vi "Main.vi"() -> ()   [LabVIEW 2019, in "Money.lvlib"]
doc: "This template is based off of the Queued Message Handler design pattern and the Queued Message Handler project template that ships with LabVIEW.\n\nThe main difference is that the queue is private to this module and communication between modules is performed via Broadcast and Request events.\n\nRequest events are wrapped in public API methods and are handled in the Event Handling Loop (EHL) of this VI. Any module can register for Broadcast events sent by this module. The EHL generates messages based on user interface actions.\n\nThe Message Handling Loop (MHL) processes messages generated by the EHL, or by other messages. The messages are string values, so new messages can be added easily to the Message Cases case structure in the MHL. Each message cluster can also provide an optional value for Message Data, which is a variant that can be converted to whatever message-specific data is required.\n_____\nBased on Delacor QMH Project Template 4.2.1.64."
uses:
  Money.lvlib
  <vilib>/Delacor/Delacor QMH/Libraries/Module Admin_class/Delacor_lib_QMH_Module Admin.lvclass
  Module Data--cluster.ctl
  <vilib>/Delacor/Delacor QMH/Libraries/Message Queue_class/Delacor_lib_QMH_Message Queue.lvclass/Delacor_lib_QMH_Message Queue.ctl
  Stop Argument--cluster.ctl
  <vilib>/Delacor/Delacor QMH/Libraries/Module Admin_class/Delacor_lib_QMH_Module Admin.lvclass/Delacor_lib_QMH_Module Admin.ctl
  Add to Balance Argument--cluster.ctl
  Add to Balance (Reply Payload)--cluster.ctl
  Refund Money Argument--cluster.ctl
  Check Funds Argument--cluster.ctl
  Check Funds (Reply Payload)--cluster.ctl
  Reduce Funds Argument--cluster.ctl
  Reduce Funds (Reply Payload)--cluster.ctl
  <vilib>/Utility/miscctls.llb/LVPointTypeDef.ctl
  <vilib>/Delacor/Delacor QMH/Libraries/Message Queue_class/Delacor_lib_QMH_Enqueue Message (Single).vi
  <vilib>/Delacor/Delacor QMH/Libraries/Module Admin_class/Delacor_lib_QMH_Get External Launch.vi
  <vilib>/Utility/error.llb/Error Cluster From Error Code.vi
  <vilib>/ErrorRing/Error Ring.xnode
  <vilib>/Delacor/Delacor QMH/Libraries/Message Queue_class/Delacor_lib_QMH_Message Queue.lvclass
panel:
  in  "Subpanel Ref":refnum<vi>
  in  "Money":T1
  in  "Simulate MHL Error":bool
  in  "Simulate EHL Error":bool
  out "error out":errorcluster
  in  "Module Admin":refnum<class "Delacor_lib_QMH_Module Admin.lvclass">
  out "Status":string
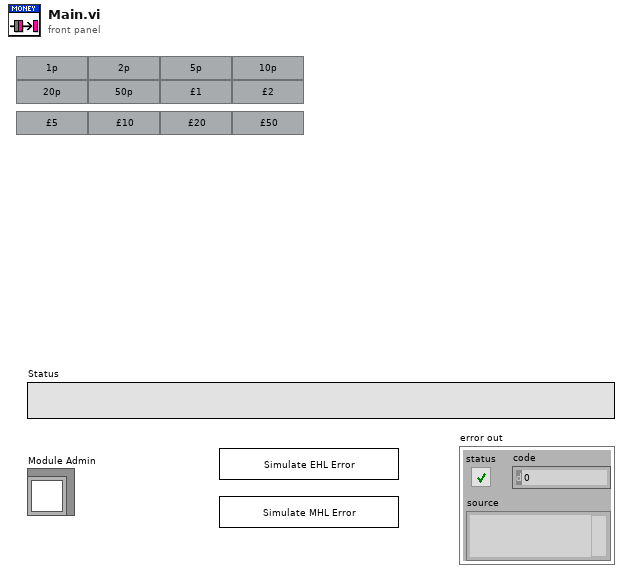
[diagram p1: front panel]
types:
  T1 = cluster{"1":bool, "2":bool, "5":bool, "10":bool, "20":bool, "50":bool, "100":bool, "200":bool, "500":bool, "1000":bool, "2000":bool, "5000":bool}
  T2 = typedef "Money.lvlib/Request Events--cluster.ctl" = cluster{"Stop Module":refnum<user-event>, "Show Panel":refnum<user-event>, "Hide Panel":refnum<user-event>, "Get Module Execution Status":refnum<user-event>, "Show Diagram":refnum<user-event>, "Refund Money":refnum<user-event>, "Check Funds":refnum<user-event>, "Reduce Funds":refnum<user-event>, "Add to Balance":refnum<user-event>}
  T3 = typedef "Money.lvlib/Module Data--cluster.ctl" = cluster{"Status":string, "Balance (pence)":u32}
  T4 = enum32{"invalid lock state", "Not Locked", "Locked (No Password)", "Password-protected"}
  T5 = typedef "Money.lvlib/Stop Argument--cluster.ctl" = cluster{"Origin":string, "Exit via Stop Module Req?":bool, "Wait for Module to stop?":bool}
  T6 = typedef "Money.lvlib/Add to Balance Argument--cluster.ctl" = cluster{"Balance to add":u32, "Wait Notifier":refnum<notifier>, "wait for reply":bool}
  T7 = typedef "Money.lvlib/Refund Money Argument--cluster.ctl" = cluster{"Boolean":bool}
  T8 = typedef "Money.lvlib/Check Funds Argument--cluster.ctl" = cluster{"Minimum Amount":u32, "Wait Notifier":refnum<notifier>, "wait for reply":bool}
  T9 = typedef "Money.lvlib/Reduce Funds Argument--cluster.ctl" = cluster{"Reduce Funds":i32, "Wait Notifier":refnum<notifier>, "wait for reply":bool}
  T10 = typedef "LVPointTypeDef.ctl" = cluster{"Horizontal":i16, "Vertical":i16}
  T11 = typedef "Money.lvlib/Check Funds (Reply Payload)--cluster.ctl" = cluster{"Sufficient Funds":bool, "Check Funds_error":errorcluster, "Balance":u32}
  T12 = typedef "Money.lvlib/Reduce Funds (Reply Payload)--cluster.ctl" = cluster{"Remaining Balance":u32, "Reduce Funds_error":errorcluster, "Sucessful":bool}
  T13 = typedef "Money.lvlib/Add to Balance (Reply Payload)--cluster.ctl" = cluster{"Add to Balance_error":errorcluster, "New Balance":u32}
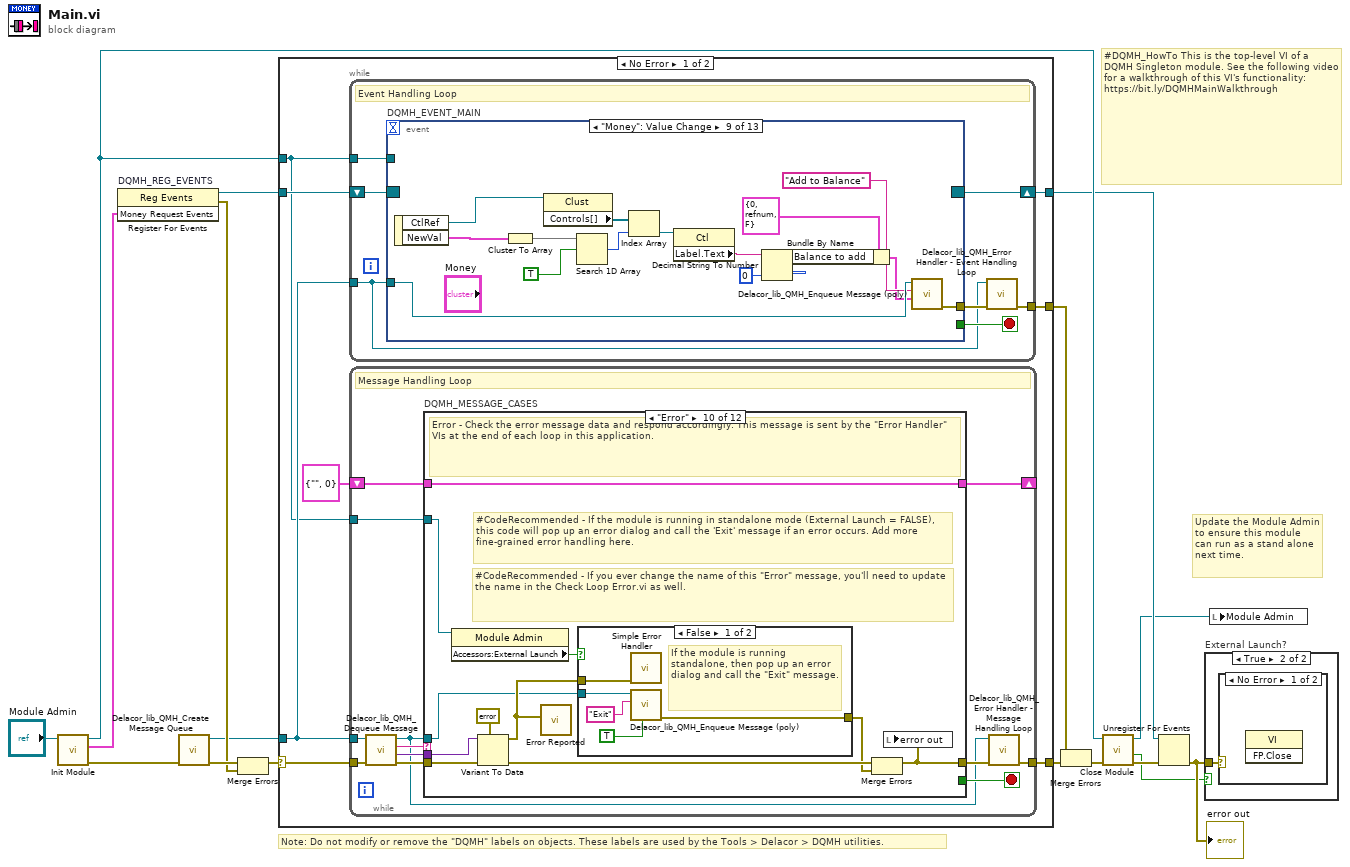
[diagram p0: block diagram]
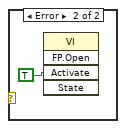
[diagram p3: hidden frame]
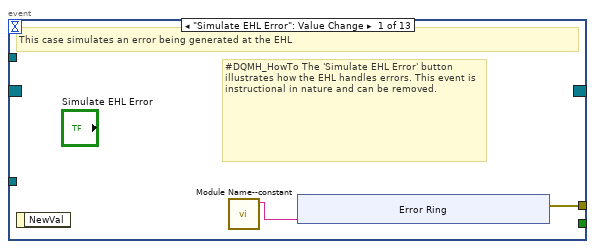
[diagram p4: hidden frame]
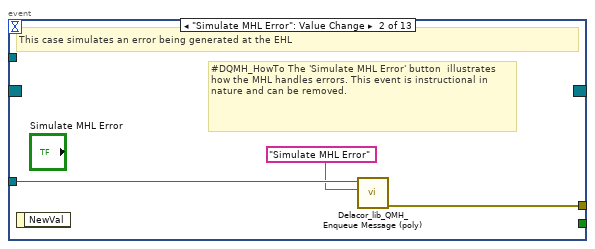
[diagram p5: hidden frame]
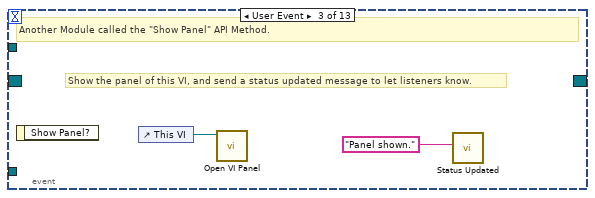
[diagram p6: hidden frame]
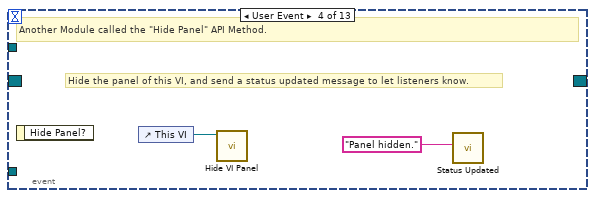
[diagram p7: hidden frame]
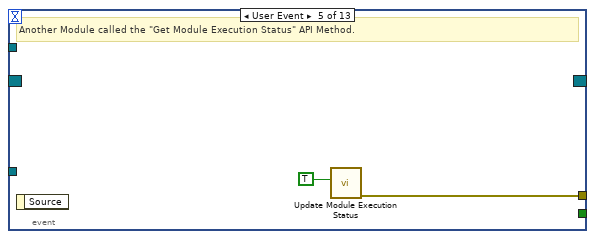
[diagram p8: hidden frame]
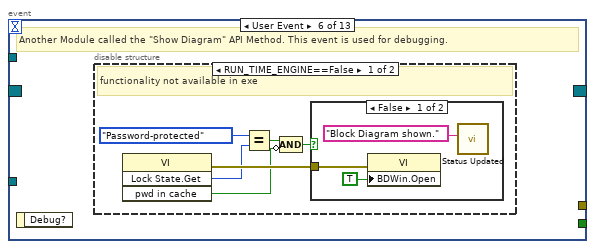
[diagram p9: hidden frame]
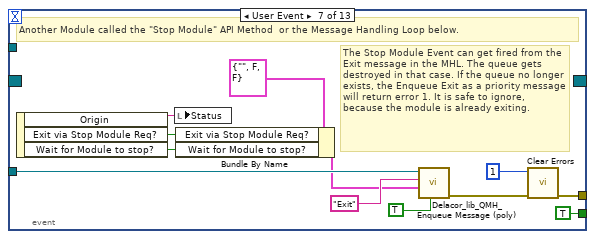
[diagram p12: hidden frame]
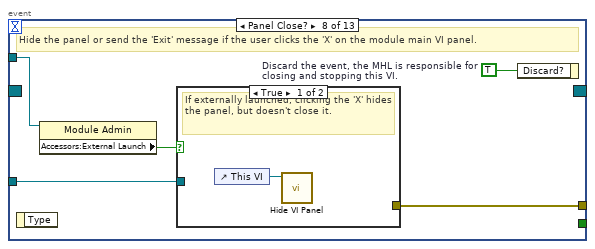
[diagram p13: hidden frame]
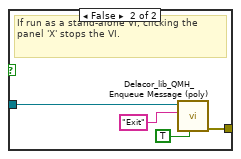
[diagram p14: hidden frame]
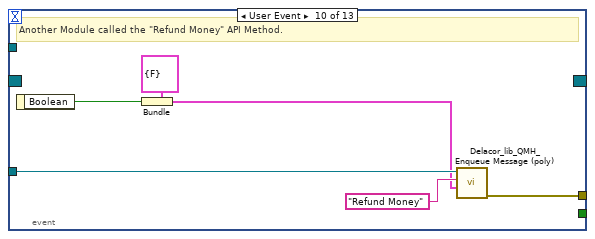
[diagram p15: hidden frame]
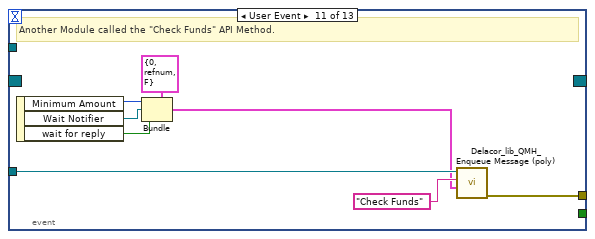
[diagram p16: hidden frame]
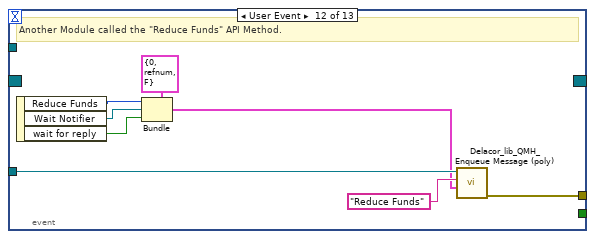
[diagram p17: hidden frame]
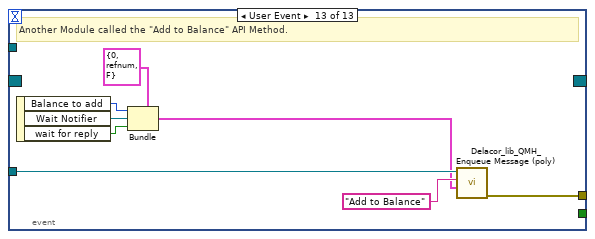
[diagram p18: hidden frame]
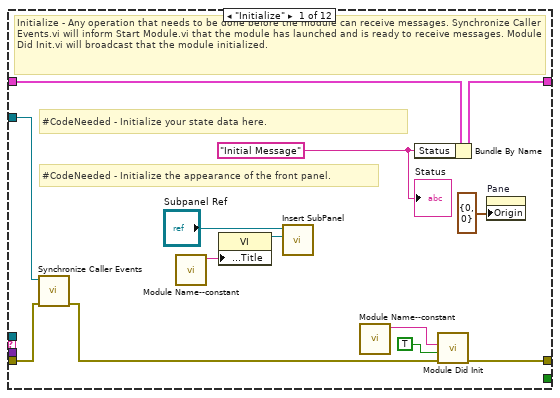
[diagram p19: hidden frame]
diagram:
  # "#DQMH_HowTo This is the top-level VI of a DQMH Singleton module. See the following video for a walkthrough of this VI's functionality: https://bit.ly/DQMHMainWalkthrough"
  # "Note: Do not modify or remove the \"DQMH\" labels on objects. These labels are used by the Tools > Delacor > DQMH utilities."
  # "Update the Module Admin to ensure this module can run as a stand alone next time."
  n1 = call "Init Module.vi"("Singleton Module Admin in"="Module Admin") -> ("error out"=w16:errorcluster, "Money Request Events"=w5:T2, "Singleton Module Admin out"=w8:refnum<class "Delacor_lib_QMH_Module Admin.lvclass">)  [unwired: 8 in]
  n2 = register-events "DQMH_REG_EVENTS"(w5) -> (reference out=w6:refnum<event-registration>, error out=w9:errorcluster)  [unwired: 2 in]
  n3 = call <vilib>:"Delacor_lib_QMH_Create Message Queue.vi"("error in (no error)"=w16) -> ("error out"=w11:errorcluster, "Message Queue"=w4:refnum<class "Delacor_lib_QMH_Message Queue.lvclass">)  [unwired: 9 in]
  n4 = Merge Errors(w11, w9) -> (w10:errorcluster)
  n5 = case shown="No Error" w10 {
    selector: w10 -> [w23 w292]
    tunnel: [w25 w292] -> w17
    tunnel: [w22 w289] -> w7
    tunnel: w6 -> [w20 w289]
    tunnel: w4 -> [w19 _]
    tunnel: [w24 _] -> w14
    tunnel: w8 -> [w18 w285]
    frame No Error {
      n6 = while {
        tunnel: w19 -> [w26]
        shift-right: [w29] -> w22
        shift-left: w20 -> [w30]
        tunnel: [w31] -> w24
        tunnel: w18 -> [w27]
        stop <- w28 stop-if-true
        # "Event Handling Loop"
        n7 = event "DQMH_EVENT_MAIN" shown="[8] \"Money\": Value Change" {
          selector: w30 -> [_ _ _ _ _ _ _ _ _ _ _ _ _]
          dyn-events: [_ _ _ _ _ _ _ _ _ _ _ _ _] -> w29
          timeout: _ -> [_ _ _ _ _ _ _ _ _ _ _ _ _]
          tunnel: [_ _ _ _ _ _ TRUE ("Discard?") _ _ _ _ _ _] -> w28
          tunnel: w26 -> [_ w43 _ _ _ _ w67 w74 w86 w102 w110 w118 w126]
          tunnel: [w34 w44 _ _ w50 _ w70 w76 w87 w97 w103 w111 w124] -> w32
          tunnel: w27 -> [_ _ _ _ _ _ _ w73 _ _ _ _ _]
          event "Simulate EHL Error": Value Change {
            # "#DQMH_HowTo The 'Simulate EHL Error' button  illustrates how the EHL handles errors. This event is instructional in nature and can be removed."
            # "This case simulates an error being generated at the EHL"
            n8 = event-data() -> ()  [unwired: 1 in, 1 out]
            n9 = call "Module Name--constant.vi"() -> ("Module Name"=w33:string)  [unwired: 11 in]
            n10 = xnode "Error Ring"("parameter 0"=w33) -> ("error out"=w34:errorcluster)
          }
          event "Simulate MHL Error": Value Change {
            # "#DQMH_HowTo The 'Simulate MHL Error' button  illustrates how the MHL handles errors. This event is instructional in nature and can be removed."
            # "This case simulates an error being generated at the EHL"
            n11 = event-data() -> ()  [unwired: 1 in, 1 out]
            n12 = call-poly <vilib>:"Delacor_lib_QMH_Enqueue Message (poly).vi"("Message"="Simulate MHL Error", "Message Queue in"=w43) -> ("error out"=w44:errorcluster)  [unwired: 8 in, 1 out]
          }
          event User Event {
            # "Show the panel of this VI, and send a status updated message to let listeners know."
            # "Another Module called the \"Show Panel\" API Method."
            n13 = event-data() -> ()  [unwired: 1 in, 1 out]
            n14 = control-ref of="This VI"() -> (w46:refnum<vi>)
            n15 = call "Open VI Panel.vi"("VI"=w46) -> ()  [unwired: 10 in, 1 out]
            n16 = call "Status Updated.vi"("Status"="Panel shown." ("format string")) -> ()  [unwired: 10 in, 1 out]
          }
          event User Event {
            # "Hide the panel of this VI, and send a status updated message to let listeners know."
            # "Another Module called the \"Hide Panel\" API Method."
            n17 = event-data() -> ()  [unwired: 1 in, 1 out]
            n18 = control-ref of="This VI"() -> (w48:refnum<vi>)
            n19 = call "Hide VI Panel.vi"("VI"=w48) -> ()  [unwired: 10 in, 1 out]
            n20 = call "Status Updated.vi"("Status"="Panel hidden." ("format string")) -> ()  [unwired: 10 in, 1 out]
          }
          event User Event {
            # "Another Module called the \"Get Module Execution Status\" API Method."
            n21 = event-data() -> ()  [unwired: 1 in, 1 out]
            n22 = call "Update Module Execution Status.vi"("Running?"=TRUE) -> ("error out"=w50:errorcluster)  [unwired: 10 in]
          }
          event User Event {
            # "Another Module called the \"Show Diagram\" API Method. This event is used for debugging."
            n23 = event-data() -> ()  [unwired: 1 in, 1 out]
            n24 = disable-structure shown="RUN_TIME_ENGINE==False" {
              frame condition #0 (active) {
                # "functionality not available in exe"
                n25 = invoke class="VI" method="Lock State.Get"() -> (error out=w56:errorcluster, "Get Lock State"=w55:T4, "pwd in cache"=w52:bool)  [unwired: 4 in, 1 out]
                n26 = Equal?(x=T4."Password-protected", y=w55) -> (x = y?=w53:bool)
                n27 = Compound Arithmetic op=AND(w53, invert w52) -> (w51:bool)
                n28 = case shown="False" w51 {
                  tunnel: w56 -> [w59 _]
                  frame False {
                    n29 = property class="VI"(error in=w59, "BDWin.Open"=TRUE ("Block Diagram Window:Open")) -> ()  [unwired: 1 in, 2 out]
                    n30 = call "Status Updated.vi"("Status"="Block Diagram shown." ("format string")) -> ()  [unwired: 10 in, 1 out]
                  }
                  frame True {
                    # "Password-protected VI, and the password is not in the cache. Do not show the diagram."
                  }
                }
              }
              frame condition #1 {
              }
            }
          }
          event User Event {
            # "The Stop Module Event can get fired from the Exit message in the MHL. The queue gets destroyed in that case. If the queue no longer exists, the Enqueue Exit as a priority message will return error 1. It is safe to ignore, because the module is already exiting."
            # "Another Module called the \"Stop Module\" API Method  or the Message Handling Loop below."
            n31 = event-data() -> ("Origin"=w66:string, "Exit via Stop Module Req?"=w62:bool, "Wait for Module to stop?"=w61:bool)  [unwired: 1 in]
            n32 = local write "Status"(w66) -> ()
            n33 = Bundle By Name(cluster=T5 {"Origin"="", "Exit via Stop Module Req?"=FALSE, "Wait for Module to stop?"=FALSE} ("Stop Argument"), "Exit via Stop Module Req?"=w62, "Wait for Module to stop?"=w61) -> (w60:T5)
            n34 = call-poly <vilib>:"Delacor_lib_QMH_Enqueue Message (poly).vi"("Priority Message? (F)"=TRUE, "Message Data"=w60, "Message"="Exit", "Message Queue in"=w67) -> ("error out"=w71:errorcluster)  [unwired: 6 in, 1 out]
            n35 = call <vilib>:"Clear Errors.vi"("error in (no error)"=w71, "specific error code to clear (0: all)"=1) -> ("error out"=w70:errorcluster)  [unwired: 4 in, 1 out]
          }
          event Panel Close? {
            w75 = TRUE  # Discard the event, the MHL is responsible for closing and stopping this VI.
            # "Hide the panel or send the 'Exit' message if the user clicks the 'X' on the module main VI panel."
            n36 = event-data() -> ()  [unwired: 1 in, 1 out]
            n37 = property class="Module Admin"(reference=w73) -> ("Accessors:External Launch"=w72:bool)  [unwired: 1 in, 2 out]
            n38 = case shown="True" w72 {
              tunnel: w74 -> [_ w80]
              tunnel: [_ w81] -> w76
              frame True {
                # "If externally launched, clicking the 'X' hides the panel, but doesn't close it."
                n39 = control-ref of="This VI"() -> (w77:refnum<vi>)
                n40 = call "Hide VI Panel.vi"("VI"=w77) -> ()  [unwired: 10 in, 1 out]
              }
              frame False {
                # "If run as a stand-alone VI, clicking the panel 'X' stops the VI."
                n41 = call-poly <vilib>:"Delacor_lib_QMH_Enqueue Message (poly).vi"("Priority Message? (F)"=TRUE, "Message"="Exit", "Message Queue in"=w80) -> ("error out"=w81:errorcluster)  [unwired: 7 in, 1 out]
              }
            }
            n42 = event-data("Discard?"=w75) -> ()  [unwired: 1 in, 1 out]
          }
          event "Money": Value Change {
            n43 = event-data() -> ("CtlRef"=w96:refnum<vi>, "NewVal"=w95:T1)  [unwired: 1 in]
            n44 = Cluster To Array(cluster=w95) -> (array=w94:bool[])
            n45 = property class="Clust"(reference=w96) -> ("Controls[]"=w88:refnum<vi>[])  [unwired: 1 in, 2 out]
            n46 = Search 1D Array(1D array=w94, element=TRUE) -> (index of element=w92:i32)  [unwired: 1 in]
            n47 = Index Array(array=w88, index=w92) -> (element=w91:refnum<vi>)
            n48 = property class="Ctl"(reference=w91) -> ("Label.Text"=w90:string)  [unwired: 1 in, 2 out]
            n49 = Decimal String To Number(string=w90, default (0L)=u32 0 ("default (0 I32)")) -> (number=w83:u32)  [unwired: 1 in, 1 out]
            n50 = Bundle By Name(cluster=T6 {"Balance to add"=0, "Wait Notifier"=refnum, "wait for reply"=FALSE} ("Add to Balance Argument"), "Balance to add"=w83) -> (w82:T6)
            n51 = call-poly <vilib>:"Delacor_lib_QMH_Enqueue Message (poly).vi"("Message Data"=w82, "Message"="Add to Balance", "Message Queue in"=w86) -> ("error out"=w87:errorcluster)  [unwired: 7 in, 1 out]
          }
          event User Event {
            # "Another Module called the \"Refund Money\" API Method."
            n52 = event-data() -> ("Boolean"=w98:bool)  [unwired: 1 in]
            n53 = Bundle(cluster=T7 {"Boolean"=FALSE} ("Refund Money Argument"), "Boolean"=w98) -> (w99:T7)
            n54 = call-poly <vilib>:"Delacor_lib_QMH_Enqueue Message (poly).vi"("Message Data"=w99, "Message"="Refund Money", "Message Queue in"=w102) -> ("error out"=w97:errorcluster)  [unwired: 7 in, 1 out]
          }
          event User Event {
            # "Another Module called the \"Check Funds\" API Method."
            n55 = event-data() -> ("Minimum Amount"=w106:u32, "Wait Notifier"=w105:refnum<notifier>, "wait for reply"=w104:bool)  [unwired: 1 in]
            n56 = Bundle(cluster=T8 {"Minimum Amount"=0, "Wait Notifier"=refnum, "wait for reply"=FALSE} ("Check Funds Argument"), "Minimum Amount"=w106, "Wait Notifier"=w105, "wait for reply"=w104) -> (w107:T8)
            n57 = call-poly <vilib>:"Delacor_lib_QMH_Enqueue Message (poly).vi"("Message Data"=w107, "Message"="Check Funds", "Message Queue in"=w110) -> ("error out"=w103:errorcluster)  [unwired: 7 in, 1 out]
          }
          event User Event {
            # "Another Module called the \"Reduce Funds\" API Method."
            n58 = event-data() -> ("Reduce Funds"=w114:i32, "Wait Notifier"=w113:refnum<notifier>, "wait for reply"=w112:bool)  [unwired: 1 in]
            n59 = Bundle(cluster=T9 {"Reduce Funds"=0, "Wait Notifier"=refnum, "wait for reply"=FALSE} ("Reduce Funds Argument"), "Reduce Funds"=w114, "Wait Notifier"=w113, "wait for reply"=w112) -> (w115:T9)
            n60 = call-poly <vilib>:"Delacor_lib_QMH_Enqueue Message (poly).vi"("Message Data"=w115, "Message"="Reduce Funds", "Message Queue in"=w118) -> ("error out"=w111:errorcluster)  [unwired: 7 in, 1 out]
          }
          event User Event {
            # "Another Module called the \"Add to Balance\" API Method."
            n61 = event-data() -> ("Balance to add"=w122:u32, "Wait Notifier"=w123:refnum<notifier>, "wait for reply"=w121:bool)  [unwired: 1 in]
            n62 = Bundle(cluster=T6 {"Balance to add"=0, "Wait Notifier"=refnum, "wait for reply"=FALSE} ("Add to Balance Argument"), "Balance to add"=w122, "Wait Notifier"=w123, "wait for reply"=w121) -> (w119:T6)
            n63 = call-poly <vilib>:"Delacor_lib_QMH_Enqueue Message (poly).vi"("Message Data"=w119, "Message"="Add to Balance", "Message Queue in"=w126) -> ("error out"=w124:errorcluster)  [unwired: 7 in, 1 out]
          }
        }
        n64 = call-dynamic "Delacor_lib_QMH_Error Handler - Event Handling Loop.vi"("error in (no error)"=w32, "Message Queue in"=w26) -> ("dup error in"=w31:errorcluster)  [unwired: 8 in, 1 out]
      }
      n65 = while {
        tunnel: w19 -> [w129]
        shift-right: [w133] -> _
        shift-left: T3 {"Status"="", "Balance (pence)"=0} ("Data Cluster") -> [w134]
        tunnel: w23 -> [w137]
        tunnel: [w135] -> w25
        tunnel: w18 -> [w127]
        stop <- w132 stop-if-true
        # "Message Handling Loop"
        n66 = call-dynamic "Delacor_lib_QMH_Dequeue Message.vi"("error in (no error)"=w137, "Message Queue in"=w129) -> ("error out"=w136:errorcluster, "Message Data"=w130:variant, "Message"=w131:string, "Message Queue out"=w128:refnum<class "Delacor_lib_QMH_Message Queue.lvclass">)  [unwired: 6 in]
        n67 = case "DQMH_MESSAGE_CASES" shown="\"Error\"" w131 {
          selector: w131 -> [_ _ _ _ _ _ _ _ _ _ _ w272]
          tunnel: w128 -> [_ _ _ _ _ _ _ _ _ w242 w264 _]
          tunnel: w136 -> [w151 w153 w164 w180 w200 w219 w225 w227 w232 w249 w270 w274]
          tunnel: [w149 w153 w157 w171 w192 w210 w224 w227 w231 w245 w267 w275] -> w138
          tunnel: w134 -> [w146 w152 w159 w170 w189 w206 w223 w226 w229 w244 w263 w273]
          tunnel: [w145 w152 w161 w170 w188 w207 w223 w226 w229 w244 w263 w273] -> w133
          tunnel: [_ _ _ _ _ _ _ _ _ _ w262 _] -> w132
          tunnel: w130 -> [_ _ w163 w178 w199 w217 _ _ _ w243 w261 _]
          tunnel: w127 -> [w147 _ _ _ _ _ _ _ _ w241 w256 _]
          frame "Initialize" {
            w141 = "Initial Message" ("Initial Message")
            # "#CodeNeeded - Initialize the appearance of the front panel."
            # "#CodeNeeded - Initialize your state data here."
            # "Initialize - Any operation that needs to be done before the module can receive messages. Synchronize Caller Events.vi will inform Start Module.vi that the module has launched and is ready to receive messages. Module Did Init.vi will broadcast that the module initialized."
            n68 = call "Synchronize Caller Events.vi"("error in (no error)"=w151, "Singleton Module Admin in"=w147) -> ("error out"=w150:errorcluster)  [unwired: 8 in, 1 out]
            n69 = call "Module Name--constant.vi"() -> ("Module Name"=w148:string)  [unwired: 11 in]
            n70 = property class="VI"("Front Panel.Title"=w148) -> (reference out=w140:refnum<vi>)  [unwired: 2 in, 1 out]
            n71 = call "Insert SubPanel.vi"("VI Ref"=w140, "Subpanel Ref"="Subpanel Ref") -> ()  [unwired: 9 in, 1 out]
            n72 = call "Module Name--constant.vi"() -> ("Module Name"=w143:string)  [unwired: 11 in]
            n73 = Bundle By Name(cluster=w146, "Status"=w141) -> (w145:T3)
            n74 = call "Module Did Init.vi"("error in (no error)"=w150, "Initialized?"=TRUE, "Origin"=w143) -> ("error out"=w149:errorcluster)  [unwired: 8 in]
            n75 = property on="Pane" class="Pane"("Origin"=T10 {"Horizontal"=0, "Vertical"=0}) -> ()  [unwired: 2 in, 2 out]
            "Status" <- w141
          }
          frame "--- Module Specific ---" {
            # "Separator -- The following cases handle messages specific to this Module."
          }
          frame "Refund Money" {
            # "Refund Money"
            n76 = Variant To Data(error in=w164, type=T7 {"Boolean"=FALSE} ("Refund Money Argument"), Variant=w163) -> (error out=w158:errorcluster)  [unwired: 1 out]
            n77 = Unbundle By Name(w159) -> ("Balance (pence)"=w156:u32)
            n78 = call "Money Refunded.vi"("error in (no error)"=w158, "Amount Refunded"=w156) -> ("error out"=w157:errorcluster)  [unwired: 9 in]
            n79 = Format Into String(format string="Money refunded: %d" ("Status"), w156) -> (resulting string=w154:string)  [unwired: 2 in, 1 out]
            n80 = Bundle By Name(cluster=w159, "Balance (pence)"=u32 0) -> (w161:T3)
            n81 = call "Status Updated.vi"("Status"=w154) -> ()  [unwired: 10 in, 1 out]
          }
          frame "Check Funds" {
            # "Check the operator has entered enough money."
            n82 = Variant To Data(error in=w180, type=T8 {"Minimum Amount"=0, "Wait Notifier"=refnum, "wait for reply"=FALSE} ("Check Funds Argument"), Variant=w178) -> (data=w176:T8, error out=w179:errorcluster)
            n83 = Unbundle By Name(w170) -> ("Balance (pence)"=w165:u32)
            n84 = Unbundle By Name(w176) -> ("Minimum Amount"=w169:u32, "Wait Notifier"=w175:refnum<notifier>, "wait for reply"=w174:bool)
            n85 = Greater Or Equal?(x=w165, y=w169) -> (x >= y?=w166:bool)
            n86 = Merge Errors(w179) -> (w171:errorcluster)
            n87 = Format Into String(format string="Checking funds. Funds %d, Sufficent: %b", w165, w166) -> (resulting string=w168:string)  [unwired: 2 in, 1 out]
            n88 = Bundle By Name(cluster=T11 {"Sufficient Funds"=FALSE, "Check Funds_error"={"status"=FALSE, "code"=0, "source"=""}, "Balance"=0} ("Check Funds (Reply Payload)"), "Balance"=w165, "Sufficient Funds"=w166) -> (w173:T11)
            n89 = call "Status Updated.vi"("Status"=w168) -> ()  [unwired: 10 in, 1 out]
            n90 = case shown="True" w174 {
              tunnel: w175 -> [_ w182]
              tunnel: w173 -> [_ w181]
              frame False {
              }
              frame True {
                n91 = Send Notification(notification=w181, notifier=w182) -> ()  [unwired: 1 in, 2 out]
              }
            }
          }
          frame "Reduce Funds" {
            # "Reduce Funds"
            n92 = Variant To Data(error in=w200, type=T9 {"Reduce Funds"=0, "Wait Notifier"=refnum, "wait for reply"=FALSE} ("Reduce Funds Argument"), Variant=w199) -> (data=w197:T9, error out=w187:errorcluster)
            n93 = Unbundle By Name(w197) -> ("Reduce Funds"=w191:i32, "Wait Notifier"=w196:refnum<notifier>, "wait for reply"=w195:bool)
            n94 = call "Reduce Funds and Check.vi"("error in (no error)"=w187, "Amount to Reduce"=w191, "Data Cluster"=w189) -> ("error out"=w186:errorcluster, "Remaining Balance"=w183:u32, "Sucessful"=w190:bool, "Data Cluster Out"=w188:T3)  [unwired: 5 in]
            n95 = Merge Errors(w186) -> (w192:errorcluster)
            n96 = Bundle By Name(cluster=T12 {"Remaining Balance"=0, "Reduce Funds_error"={"status"=FALSE, "code"=0, "source"=""}, "Sucessful"=FALSE} ("Reduce Funds (Reply Payload)"), "Sucessful"=w190, "Remaining Balance"=w183) -> (w194:T12)
            n97 = Format Into String(format string="Reducing Funds. Balance: %d", w183) -> (resulting string=w184:string)  [unwired: 2 in, 1 out]
            n98 = call "Status Updated.vi"("Status"=w184) -> ()  [unwired: 10 in, 1 out]
            n99 = case shown="True" w195 {
              tunnel: w196 -> [_ w202]
              tunnel: w194 -> [_ w201]
              frame False {
              }
              frame True {
                n100 = Send Notification(notification=w201, notifier=w202) -> ()  [unwired: 1 in, 2 out]
              }
            }
          }
          frame "Add to Balance" {
            n101 = Variant To Data(error in=w219, type=T6 {"Balance to add"=0, "Wait Notifier"=refnum, "wait for reply"=FALSE} ("Add to Balance Argument"), Variant=w217) -> (data=w215:T6, error out=w218:errorcluster)
            n102 = Unbundle By Name(w206) -> ("Balance (pence)"=w209:u32)
            n103 = Unbundle By Name(w215) -> ("Balance to add"=w208:u32, "Wait Notifier"=w214:refnum<notifier>, "wait for reply"=w213:bool)
            n104 = Add(x=w209, y=w208) -> (x+y=w203:u32)
            n105 = Bundle By Name(cluster=w206, "Balance (pence)"=w203) -> (w207:T3)
            n106 = Merge Errors(w218) -> (w210:errorcluster)
            n107 = Format Into String(format string="Added Funds. Balance: %d", w203) -> (resulting string=w204:string)  [unwired: 2 in, 1 out]
            n108 = Bundle By Name(cluster=T13 {"Add to Balance_error"={"status"=FALSE, "code"=0, "source"=""}, "New Balance"=0} ("Add to Balance (Reply Payload)"), "New Balance"=w203) -> (w212:T13)
            n109 = call "Status Updated.vi"("Status"=w204) -> ()  [unwired: 10 in, 1 out]
            n110 = case shown="False" w213 {
              tunnel: w214 -> [_ w222]
              tunnel: w212 -> [_ w221]
              tunnel: w203 -> [w220 _]
              frame False {
                n111 = call "Money Entered.vi"("New Balance"=w220) -> ()  [unwired: 10 in, 1 out]
              }
              frame True {
                n112 = Send Notification(notification=w221, notifier=w222) -> ()  [unwired: 1 in, 2 out]
              }
            }
          }
          frame "---Copy This Frame---" {
            # "Duplicate this frame when creating new messages.  Change this comment in the duplicated frame to describe this message."
            n113 = Merge Errors(w225) -> (w224:errorcluster)
          }
          frame "--- Exit and Error Handling---" {
            # "Separator - The following cases handle errors and exit messages."
          }
          frame "Simulate MHL Error" {
            # "#DQMH_HowTo The 'Simulate MHL Error' button  illustrates how the MHL handles errors. This event is instructional in nature and can be removed."
            # "Simulate an error occurring at the MHL"
            n114 = call "Module Name--constant.vi"() -> ("Module Name"=w228:string)  [unwired: 11 in]
            n115 = xnode "Error Ring"("parameter 0"=w228) -> ("error out"=w230:errorcluster)
            n116 = Merge Errors(w232, w230) -> (w231:errorcluster)
          }
          frame "Error" {
            # "#CodeRecommended - If you ever change the name of this \"Error\" message, you'll need to update the name in the Check Loop Error.vi as well."
            # "#CodeRecommended - If the module is running in standalone mode (External Launch = FALSE), this code will pop up an error dialog and call the 'Exit' message if an error occurs. Add more fine-grained error handling here."
            # "Error - Check the error message data and respond accordingly. This message is sent by the \"Error Handler\" VIs at the end of each loop in this application."
            n117 = property class="Module Admin"(reference=w241) -> ("Accessors:External Launch"=w240:bool)  [unwired: 1 in, 2 out]
            n118 = Variant To Data(error in=w249, type=errorcluster {"status"=FALSE, "code"=0, "source"=""} ("error constant"), Variant=w243) -> (data=w250:errorcluster, error out=w247:errorcluster)
            n119 = call "Error Reported.vi"("Error"=w250) -> ()  [unwired: 10 in, 1 out]
            n120 = case shown="False" w240 {
              tunnel: [w255 _] -> w246
              tunnel: w242 -> [w253 _]
              tunnel: w250 -> [w254 _]
              frame False {
                # "If the module is running standalone, then pop up an error dialog and call the \"Exit\" message."
                n121 = call <vilib>:"Simple Error Handler.vi"("error in (no error)"=w254) -> ()  [unwired: 4 in, 5 out]
                n122 = call-poly <vilib>:"Delacor_lib_QMH_Enqueue Message (poly).vi"("Priority Message? (F)"=TRUE, "Message"="Exit", "Message Queue in"=w253) -> ("error out"=w255:errorcluster)  [unwired: 7 in, 1 out]
              }
              frame True {
                # "If the module was launched externally, calling the Error Reported broadcast VI is the only action performed by the \"Error\" message. The module's caller can then process the error appropriately."
              }
            }
            n123 = Merge Errors(w247, w246) -> (w245:errorcluster)
            n124 = local write "error out"(w245) -> ()
          }
          frame "Exit" {
            w260 = 91  # 91: not all Exit messages will have an argument
            w262 = TRUE  # Stop the VI
            # "Release the message queue reference"
            # "#CodeNeeded - Add any required cleanup code here"
            # "Exit - Exit the application."
            n125 = Variant To Data(error in=w270, type=T5 {"Origin"="", "Exit via Stop Module Req?"=FALSE, "Wait for Module to stop?"=FALSE} ("Stop Argument"), Variant=w261) -> (data=w258:T5, error out=w266:errorcluster)
            n126 = call <vilib>:"Clear Errors.vi"("error in (no error)"=w266, "specific error code to clear (0: all)"=w260) -> ("error out"=w269:errorcluster)  [unwired: 4 in, 1 out]
            n127 = control-ref of="This VI"() -> (w257:refnum<vi>)
            n128 = call-dynamic "Delacor_lib_QMH_Release Message Queue.vi"("error in (no error)"=w269, "Message Queue"=w264) -> ("error out"=w268:errorcluster)  [unwired: 9 in]
            n129 = call "Handle Exit.vi"("Stop Argument"=w258, "Admin in"=w256, "VI reference"=w257) -> ("error out"=w265:errorcluster)  [unwired: 7 in, 1 out]
            n130 = Merge Errors(w268, w265) -> (w267:errorcluster)
          }
          frame Default {
            # "'Default' case only runs if there is a message that isn't defined in any of the other cases.  Output a programming error."
            n131 = call "Module Name--constant.vi"() -> ("Module Name"=w271:string)  [unwired: 11 in]
            n132 = xnode "Error Ring"("parameter 0"=w272, "parameter 1"=w271) -> ("error out"=w276:errorcluster)
            n133 = Merge Errors(w274, w276) -> (w275:errorcluster)
          }
        }
        n134 = call-dynamic "Delacor_lib_QMH_Error Handler - Message Handling Loop.vi"("error in (no error)"=w138, "Message Queue in"=w128) -> ("dup error in"=w135:errorcluster)  [unwired: 8 in, 1 out]
      }
    }
    frame Error {
      # "Synchronize Caller Events.vi will inform Start Module.vi that the module has launched and will let the code calling Start Module.vi register for broadcasts and would permit the caller receive the broadcast that an error occurred at launch time."
      n135 = call "Synchronize Caller Events.vi"("Singleton Module Admin in"=w285) -> ("error out"=w290:errorcluster)  [unwired: 9 in, 1 out]
      n136 = call "Module Name--constant.vi"() -> ("Module Name"=w288:string)  [unwired: 11 in]
      n137 = Format Into String(format string="An error occurred during initialization. %s is no longer running.", w288) -> (resulting string=w286:string)  [unwired: 2 in, 1 out]
      n138 = Merge Errors(w292, w290) -> (w291:errorcluster)
      n139 = call "Error Reported.vi"("Additional Information"=w286, "Error"=w291) -> ()  [unwired: 9 in, 1 out]
    }
  }
  n140 = Merge Errors(w14, w17) -> (w13:errorcluster)
  n141 = call "Close Module.vi"("error in (no error)"=w13, "Module Admin in"=w8) -> ("error out"=w15:errorcluster, "External Launch"=w1:bool, "Module Admin out"=w2:refnum<class "Delacor_lib_QMH_Module Admin.lvclass">)  [unwired: 7 in]
  n142 = Unregister For Events(event registration refnum=w7, error in=w15) -> (error out=w12:errorcluster)
  "error out" <- w12
  n143 = case "External Launch?" shown="True" w1 {
    tunnel: w12 -> [_ w293]
    frame False {
    }
    frame True {
      n144 = case shown="No Error" w293 {
        frame No Error {
          n145 = invoke class="VI" method="FP.Close"() -> ()  [unwired: 3 in, 3 out]
        }
        frame Error {
          n146 = invoke class="VI" method="FP.Open"("Activate"=TRUE ("Activate?")) -> ()  [unwired: 4 in, 5 out]
        }
      }
    }
  }
  n147 = local write "Module Admin"(w2) -> ()
